vi "Write Gobject.vi"(3 "GObject_FPSZ":refnum<class "GObject_FPSZ.lvclass">, 4 "GObj":refnum<vi>) -> (5 "GObject_FPSZ Out":refnum<class "GObject_FPSZ.lvclass">)   [LabVIEW 2023, in "GObject_FPSZ.lvclass"]
uses:
  GObject_FPSZ.lvclass
  GObject_FPSZ.lvclass/GObject_FPSZ.ctl
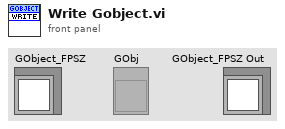
[diagram p1: front panel]
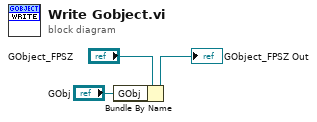
[diagram p0: block diagram]
diagram:
  n1 = Bundle By Name(cluster="GObject_FPSZ", "GObj"="GObj") -> (→"GObject_FPSZ Out":refnum<class "GObject_FPSZ.lvclass">)
